vi "OpenResourceByName.vi"   [LabVIEW 2014, in "LVFPGAAdvSessionResources.lvlib"]
uses:
  LVFPGAAdvSessionResources.lvlib
  OpenByNameSubVI.vi
  <vilib>/Utility/error.llb/Error Cluster From Error Code.vi
  <vilib>/rvi/interface/common/dynamic/niFpgaEscapeDelimiterAndNull.vi
  OpenByName.xnode
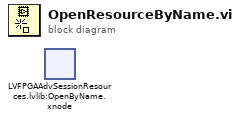
[diagram p0: block diagram]
diagram:
  n1 = xnode "LVFPGAAdvSessionResources.lvlib:OpenByName.xnode"() -> ()  [unwired: 4 in, 3 out]
